vi "Initialize with Options.vi"(7 "Option string (\"\")":string, 8 "error in (no error)":errorcluster, 9 "Reset (T: Reset)":bool=TRUE, 10 "ID Query (T: Check)":bool=TRUE, 11 "VISA resource name":refnum<visa-resource-name>) -> (0 "error out":errorcluster, 3 "VISA resource name out":refnum<visa-resource-name>)   [LabVIEW 2020, in "Rohde&Schwarz RTx Oscilloscopes.lvlib"]
doc: "This VI opens a new session to the instrument.\nCompared to the <b>Initialize.vi</b>, this one allows for additional settings in the <b>Option string</b>."
uses:
  Rohde&Schwarz RTx Oscilloscopes.lvlib
  type_Session_Parameter_int32.ctl
  type_Session_Parameter_Boolean.ctl
  type_AdditionalFlag_Bits.ctl
  rsidr_core_global.vi
  rsidr_core.lvlib
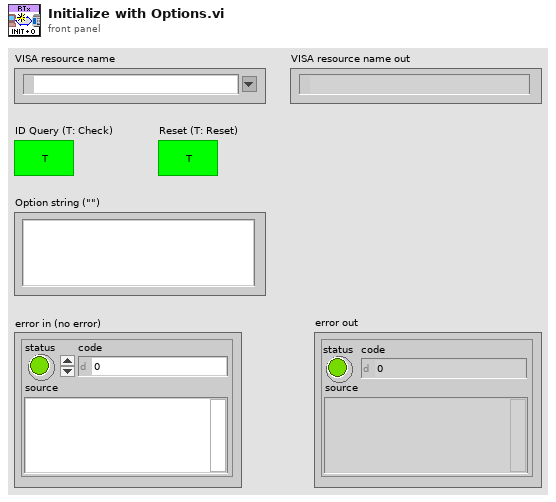
[diagram p1: front panel]
types:
  T1 = typedef "Rohde&Schwarz RTx Oscilloscopes.lvlib/rsidr_core.lvlib/type_AdditionalFlag_Bits.ctl" = enum16{"Send LF after Bin Block", "Junk read with io_clear_buffers.vi", "io_clear_buffers: viClear()", "io_clear_buffers: viFlush()", "<NotUsed1>", "Allow Dbl & Int Bin/Ascii read", "*OPC? in check_instrument_error.vi", "<NotUsed2>", "Smart Enum Matching", "Less Strict RepCaps check", "AssureResponseEndWithLF"}
  T2 = typedef "Rohde&Schwarz RTx Oscilloscopes.lvlib/rsidr_core.lvlib/type_Session_Parameter_Boolean.ctl" = enum16{"Simulate", "Query Instr Status", "Check Range", "Check Options", "Add LF to Write", "Duplicate Session", "Fast Sweep", "Logging", "OPC-sync Attribute Queries", "OPC-sync Attribute Writes"}
  T3 = typedef "Rohde&Schwarz RTx Oscilloscopes.lvlib/rsidr_core.lvlib/type_Session_Parameter_int32.ctl" = enum16{"OPC Timeout", "Additional Flags", "Wait Before Write", "Wait Before Read", "Bin Data Chunk Size", "VISA Access Mode", "VISA Timeout", "Bin Float Number Format", "Bin Integer Number Format", "STBpollVISAtimeout", "OPCwaitMode"}
  T4 = typedef "Rohde&Schwarz RTx Oscilloscopes.lvlib/rsidr_core.lvlib/type_Input_Format_RepCap.ctl" = cluster{"repCapName":string, "indetifiers":string[], "cmdValues":string[]}
  T5 = typedef "Rohde&Schwarz RTx Oscilloscopes.lvlib/rsidr_core.lvlib/type_Input_Format_RangeTable.ctl" = cluster{"Type":u16, "Name":string, "Entries":cluster{"Name":string, "Value 1":dbl, "Value 2":dbl, "Command":string}[]}
  T6 = typedef "Rohde&Schwarz RTx Oscilloscopes.lvlib/rsidr_core.lvlib/type_Input_Format_Attribute.ctl" = cluster{"Level":i32, "Class Only":bool, "Identifier":string, "Descriptive Name":string, "Data Type":u16, "Command":string, "Access":u16, "Range Table":string, "Read Callback":string, "Write Callback":string, "Supported Models":string, "Instrument Options":string, "Flags":i32, "Help":string}
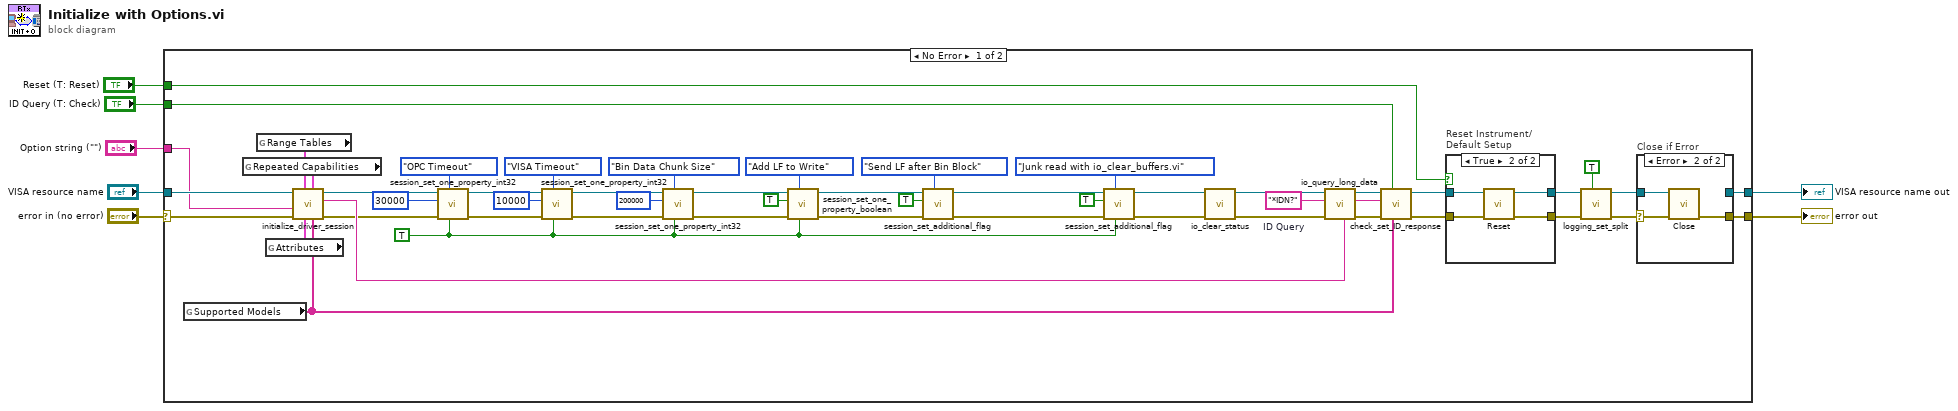
[diagram p0: block diagram]
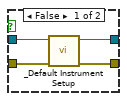
[diagram p3: hidden frame]
diagram:
  n1 = case shown="No Error" "error in (no error)" {
    selector: "error in (no error)" -> [w51 w73]
    tunnel: [w59 _] -> w7
    tunnel: [w52 w73] -> w6
    tunnel: "VISA resource name" -> [w50 _]
    tunnel: "Option string (\"\")" -> [w39 _]
    tunnel: "Reset (T: Reset)" -> [w38 _]
    tunnel: "ID Query (T: Check)" -> [w37 _]
    frame No Error {
      w10 = TRUE ("Skip setting if in option string (F)")
      w53 = "*IDN?"  # ID Query
      n2 = global read "rsidr_core_global.vi" "Supported Models"() -> (w44:string[])
      n3 = global read "rsidr_core_global.vi" "Repeated Capabilities"() -> (w41:T4[])
      n4 = global read "rsidr_core_global.vi" "Range Tables"() -> (w42:T5[])
      n5 = global read "rsidr_core_global.vi" "Attributes"() -> (w43:T6[])
      n6 = call "initialize_driver_session.vi"("Supported instruments"=w44, "Repeated Capabilities"=w41, "Attributes"=w43, "Range Tables"=w42, "error in"=w51, "Option String"=w39, "VISA resource name"=w50) -> ("error out"=w24:errorcluster, "Simulation *IDN? response out"=w40:string, "VISA resource name out"=w23:refnum<visa-resource-name>)  [unwired: 2 in]
      n7 = call "session_set_one_property_int32.vi"("Skip setting if in Options string (F)"=w10, "Session Parameter Integer"=type_Session_Parameter_int32."OPC Timeout" ("Session Parameter to set"), "error in"=w24, "Int32 value in"=30000 ("OPC Timeout"), "VISA resource name"=w23) -> ("error out"=w22:errorcluster, "VISA resource name out"=w21:refnum<visa-resource-name>)  [unwired: 4 in, 1 out]
      n8 = call "session_set_one_property_int32.vi"("Skip setting if in Options string (F)"=w10, "Session Parameter Integer"=type_Session_Parameter_int32."VISA Timeout" ("Session Parameter to set"), "error in"=w22, "Int32 value in"=10000 ("VISA Timeout"), "VISA resource name"=w21) -> ("error out"=w28:errorcluster, "VISA resource name out"=w27:refnum<visa-resource-name>)  [unwired: 4 in, 1 out]
      n9 = call "session_set_one_property_int32.vi"("Skip setting if in Options string (F)"=w10, "Session Parameter Integer"=type_Session_Parameter_int32."Bin Data Chunk Size" ("Session Parameter to set"), "error in"=w28, "Int32 value in"=200000 ("VISA Timeout"), "VISA resource name"=w27) -> ("error out"=w26:errorcluster, "VISA resource name out"=w25:refnum<visa-resource-name>)  [unwired: 4 in, 1 out]
      n10 = call "session_set_one_property_boolean.vi"("Skip setting if in Options string (F)"=w10, "Session Parameter Boolean"=type_Session_Parameter_Boolean."Add LF to Write" ("Session Parameter boolean"), "error in"=w26, "Boolean value in"=TRUE ("boolean value in"), "VISA resource name"=w25) -> ("error out"=w19:errorcluster, "VISA resource name out"=w18:refnum<visa-resource-name>)  [unwired: 4 in, 1 out]
      n11 = call "session_set_additional_flag.vi"("AdditionalFlag Bit"=type_AdditionalFlag_Bits."Send LF after Bin Block" ("AdditionalFlag bit"), "error in"=w19, "New value in"=TRUE, "VISA resource name"=w18) -> ("error out"=w12:errorcluster, "VISA resource name out"=w11:refnum<visa-resource-name>)  [unwired: 5 in, 1 out]
      n12 = call "session_set_additional_flag.vi"("Skip setting if in Options string (F)"=w10, "AdditionalFlag Bit"=type_AdditionalFlag_Bits."Junk read with io_clear_buffers.vi" ("AdditionalFlag bit"), "error in"=w12, "New value in"=TRUE, "VISA resource name"=w11) -> ("error out"=w9:errorcluster, "VISA resource name out"=w8:refnum<visa-resource-name>)  [unwired: 4 in, 1 out]
      n13 = call "io_clear_status.vi"("error in"=w9, "VISA resource name"=w8) -> ("error out"=w36:errorcluster, "VISA resource name out"=w35:refnum<visa-resource-name>)  [unwired: 8 in]
      n14 = call "io_query_long_data.vi"("Simulation read buffer (\"Simulation\")"=w40, "error in"=w36, "write buffer"=w53, "VISA resource name"=w35) -> ("error out"=w56:errorcluster, "read buffer"=w54:string, "VISA resource name out"=w55:refnum<visa-resource-name>)  [unwired: 5 in]
      n15 = call "check_set_ID_response.vi"("Supported instruments in"=w44, "Error if ID Query check fails"=w37, "error in"=w56, "IDN string in"=w54, "VISA resource name"=w55) -> ("error out"=w57:errorcluster, "VISA resource name out"=w58:refnum<visa-resource-name>)  [unwired: 3 in, 2 out]
      n16 = case "Reset Instrument/\nDefault Setup" shown="True" w38 {
        tunnel: w57 -> [w68 w72]
        tunnel: [w66 w71] -> w49
        tunnel: w58 -> [w67 w70]
        tunnel: [w65 w69] -> w48
        frame False {
          n17 = call "_Default Instrument Setup.vi"("error in"=w68, "VISA resource name"=w67) -> ("error out"=w66:errorcluster, "VISA resource name out"=w65:refnum<visa-resource-name>)  [unwired: 8 in]
        }
        frame True {
          n18 = call "Reset.vi"("error in (no error)"=w72, "VISA resource name"=w70) -> ("error out"=w71:errorcluster, "VISA resource name out"=w69:refnum<visa-resource-name>)  [unwired: 8 in]
        }
      }
      n19 = call "logging_set_split.vi"("Evaluate section error (F)"=TRUE, "error in"=w49, "VISA resource name"=w48) -> ("error out"=w47:errorcluster, "VISA resource name out"=w46:refnum<visa-resource-name>)  [unwired: 7 in]
      n20 = case "Close if Error" shown="Error" w47 {
        selector: w47 -> [w60 w63]
        tunnel: w46 -> [w61 w64]
        tunnel: [w61 _] -> w59
        tunnel: [w60 w62] -> w52
        frame No Error {
        }
        frame Error {
          n21 = call "Close.vi"("error in (no error)"=w63, "VISA resource name"=w64) -> ("error out"=w62:errorcluster)  [unwired: 9 in]
        }
      }
    }
    frame Error {
    }
  }
  "VISA resource name out" <- w7
  "error out" <- w6
